vi "Generate Random Numbers.vi"(11 "Quantity to Generate":i32) -> (3 "Random Numbers out":dbl[](array[numeric]))   [LabVIEW 2020, in "UIProgressUpdates.lvlib"]
uses:
  UIProgressUpdates.lvlib
  <vilib>/numeric/Random Number (Range) DBL.vi
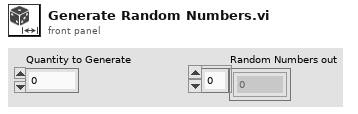
[diagram p1: front panel]
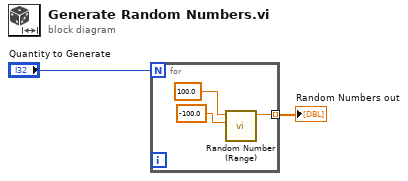
[diagram p0: block diagram]
diagram:
  n1 = for {
    N: "Quantity to Generate" -> [_]
    tunnel: [w3] -> w2 mode=indexing
    n2 = call-poly <vilib>:"Random Number (Range).vi"("lower bound (0)"=-100.0, "upper bound (100)"=100.0) -> ("number"=w3:dbl)  [unwired: 9 in]
  }
  "Random Numbers out" <- w2
